vi "Module Cleanup.vi"(8 "error in (no error)":errorcluster, 11 "GenericGuiAI in":refnum<class "GenericGuiAI.lvclass">) -> (0 "error out":errorcluster, 3 "GenericGuiAI out":refnum<class "GenericGuiAI.lvclass">)   [LabVIEW 2020, in "VolatusDAQGenericGUI.lvlib" / "GenericGuiAI.lvclass"]
uses:
  GenericGuiAI.lvclass
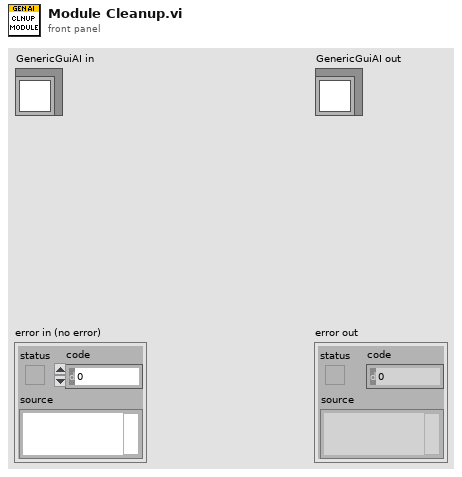
[diagram p1: front panel]
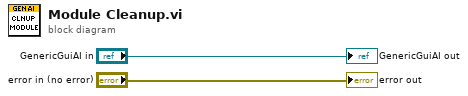
[diagram p0: block diagram]
diagram:
  "error out" <- "error in (no error)"
  "GenericGuiAI out" <- "GenericGuiAI in"
